vi "Quadrature - Linear.vi"() -> (3 "data":dbl)   [LabVIEW 2018]
uses:
  <vilib>/DAQmx/read.llb/DAQmx Read (Counter U32 1Chan 1Samp).vi
  <vilib>/DAQmx/create/channels.llb/DAQmx Create Channel (CI-Position-Linear Encoder).vi
  <vilib>/DAQmx/miscellaneous.llb/DAQmx Fill In Error Info.vi
panel:
  out "error out":errorcluster
  in  "stop":bool
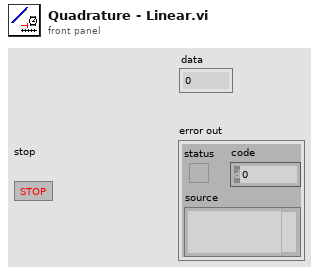
[diagram p1: front panel]
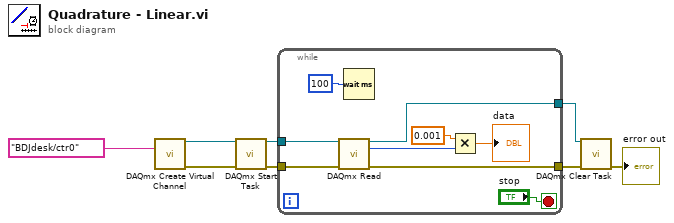
[diagram p0: block diagram]
diagram:
  n1 = call-poly <vilib>:"DAQmx Create Virtual Channel.vi"("counter"=tag "BDJdesk/ctr0") -> ("task out"=w8:refnum<k21>, "error out"=w2:errorcluster)  [unwired: 13 in]
  n2 = call <vilib>:"DAQmx Start Task.vi"("task/channels in"=w8, "error in"=w2) -> ("task out"=w7:refnum<k21>, "error out"=w5:errorcluster)  [unwired: 12 in]
  n3 = while {
    tunnel: w7 -> [w16]
    tunnel: [w15] -> w4
    tunnel: w5 -> [w10]
    tunnel: [w9] -> w1
    stop <- "stop" stop-if-true
    n4 = call-poly <vilib>:"DAQmx Read.vi"("task/channels in"=w16, "error in"=w10) -> ("task out"=w15:refnum<k21>, "data"=w14:u32, "error out"=w9:errorcluster)  [unwired: 11 in]
    n5 = Wait (ms)(milliseconds to wait=u32 100) -> ()  [unwired: 1 out]
    n6 = Multiply(x=0.001, y=w14) -> (x*y=→"data":dbl)
  }
  n7 = call <vilib>:"DAQmx Clear Task.vi"("task in"=w4, "error in"=w1) -> ("error out"=→"error out":errorcluster)  [unwired: 13 in]
